vi "uc480_SimpleLive_MultiCamera.vi"() -> ()   [LabVIEW 2015]
uses:
  C:/Program Files/Thorlabs/Scientific Imaging/DCx Camera Support/Develop/DotNet/uc480DotNet.dll
panel:
  out "Image Out":T1(plugin-control)
  in  "Init Camera 2":bool
  in  "Exit Camera 2":bool
  out "Error Out 2":errorcluster caption="error"
  out "Bits/Pixel 2":i32=8
  out "Width":i32=8
  out "Height Height 2":i32=8
  out "Serial Number 2":string
  in  "Camera ID 2":i32
  out "Image second camera":picture
  out "Image first camera":picture
  in  "Camera ID 1":i32
  out "Serial Number 1":string
  out "Height Height":i32=8
  out "Width":i32=8
  out "Bits/Pixel":i32=8
  out "Error Out 1":errorcluster caption="error"
  in  "Exit Camera":bool
  in  "Init Camera":bool
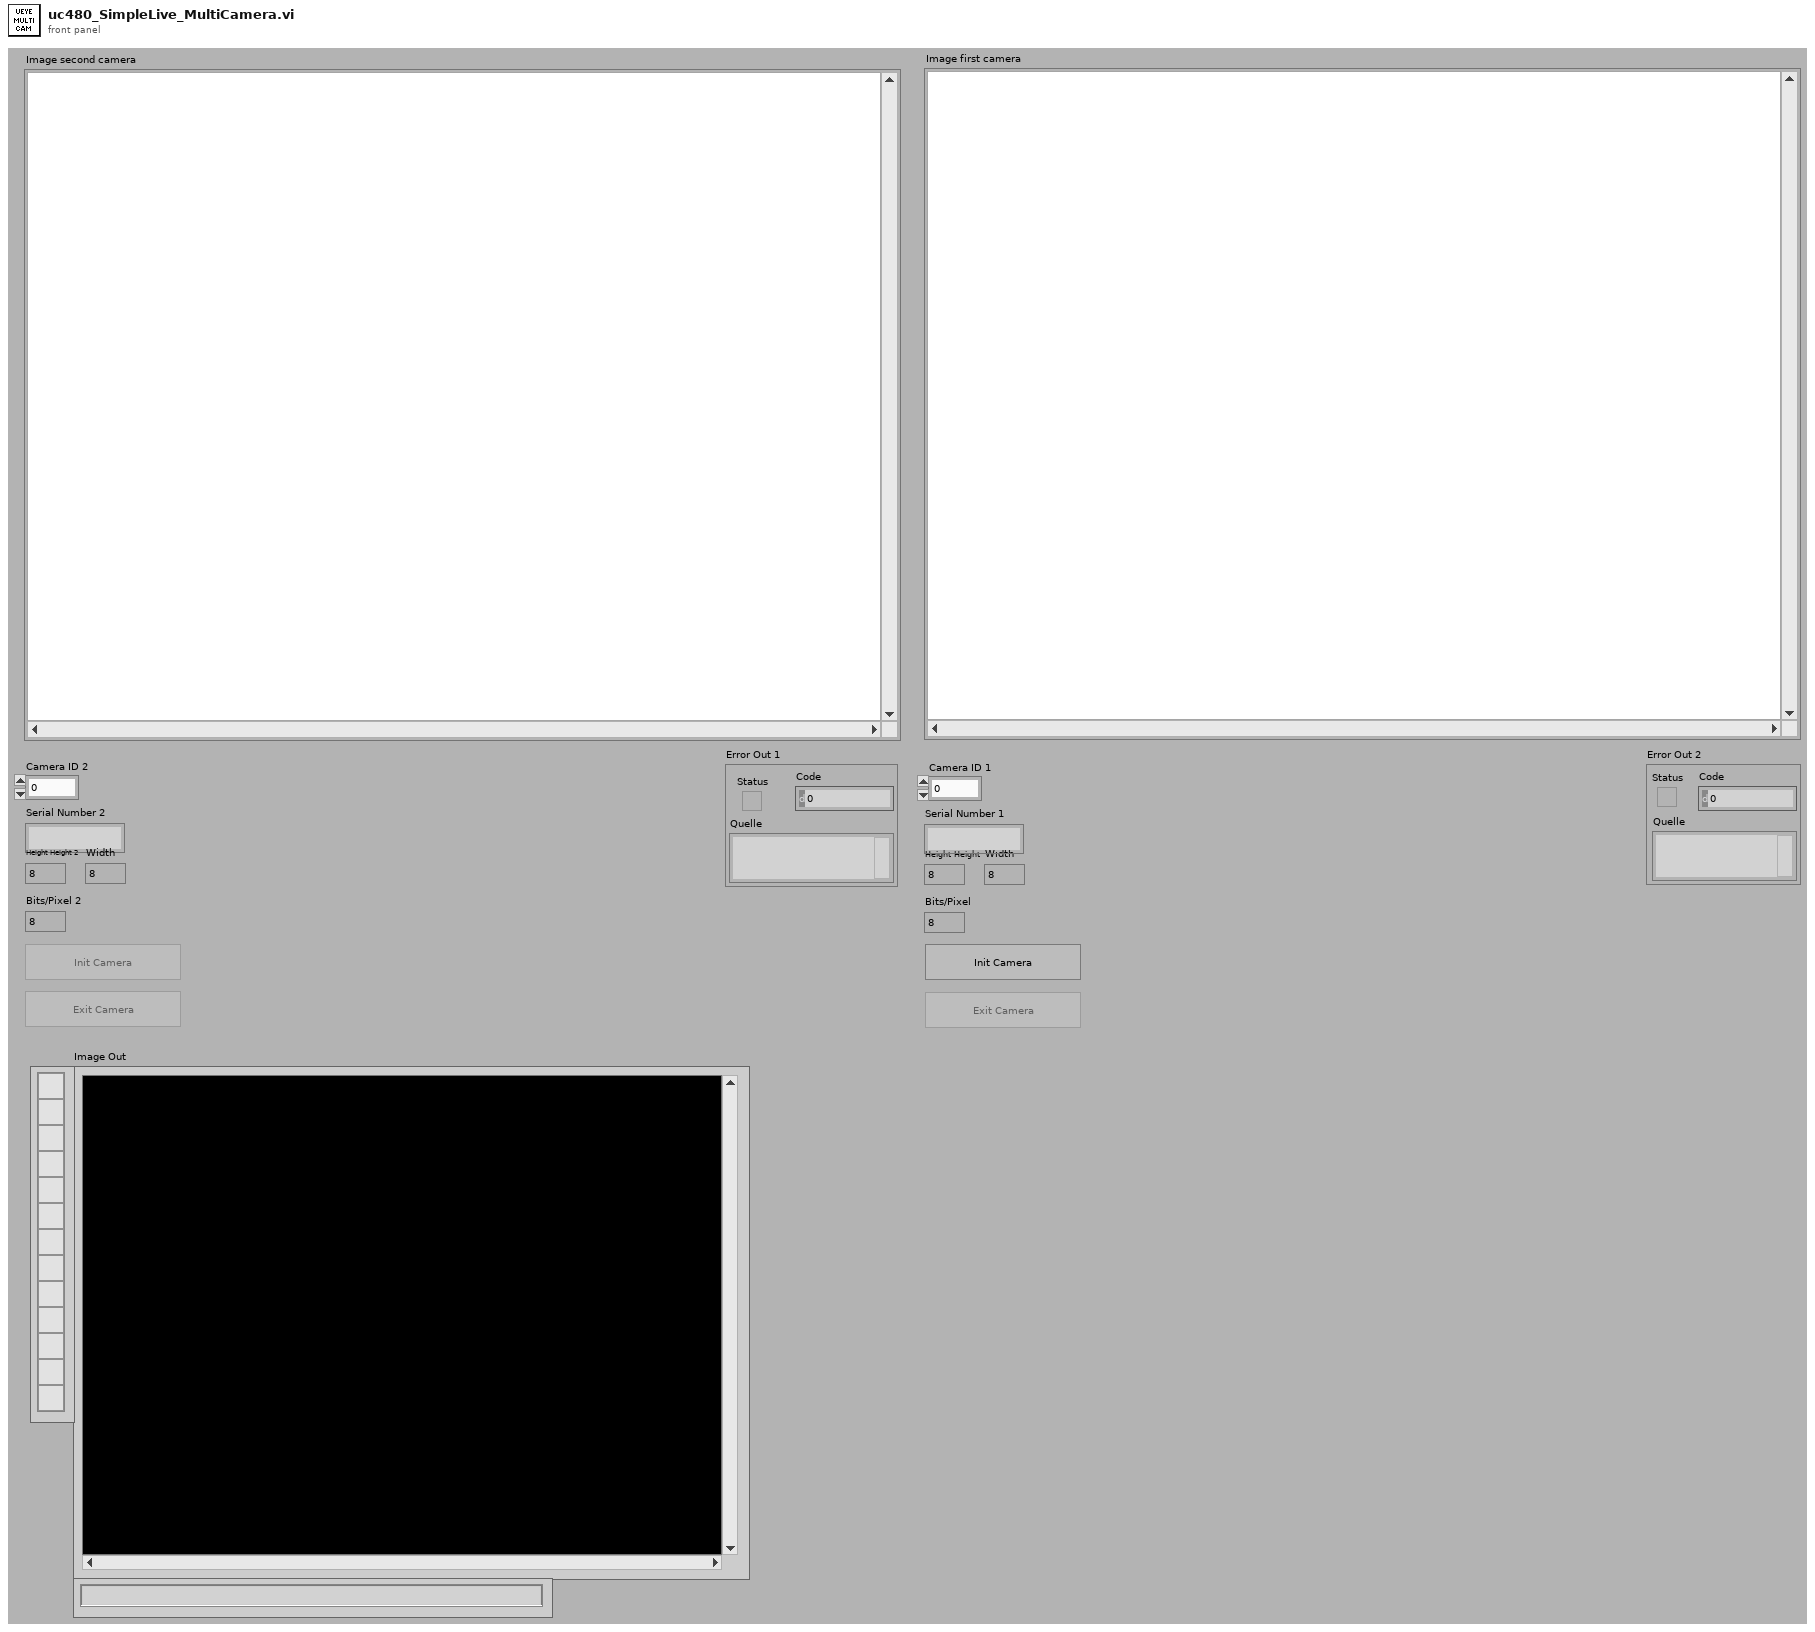
[diagram p1: front panel]
types:
  T1 = typedef "IMAQ Image.ctl" = refnum<image>
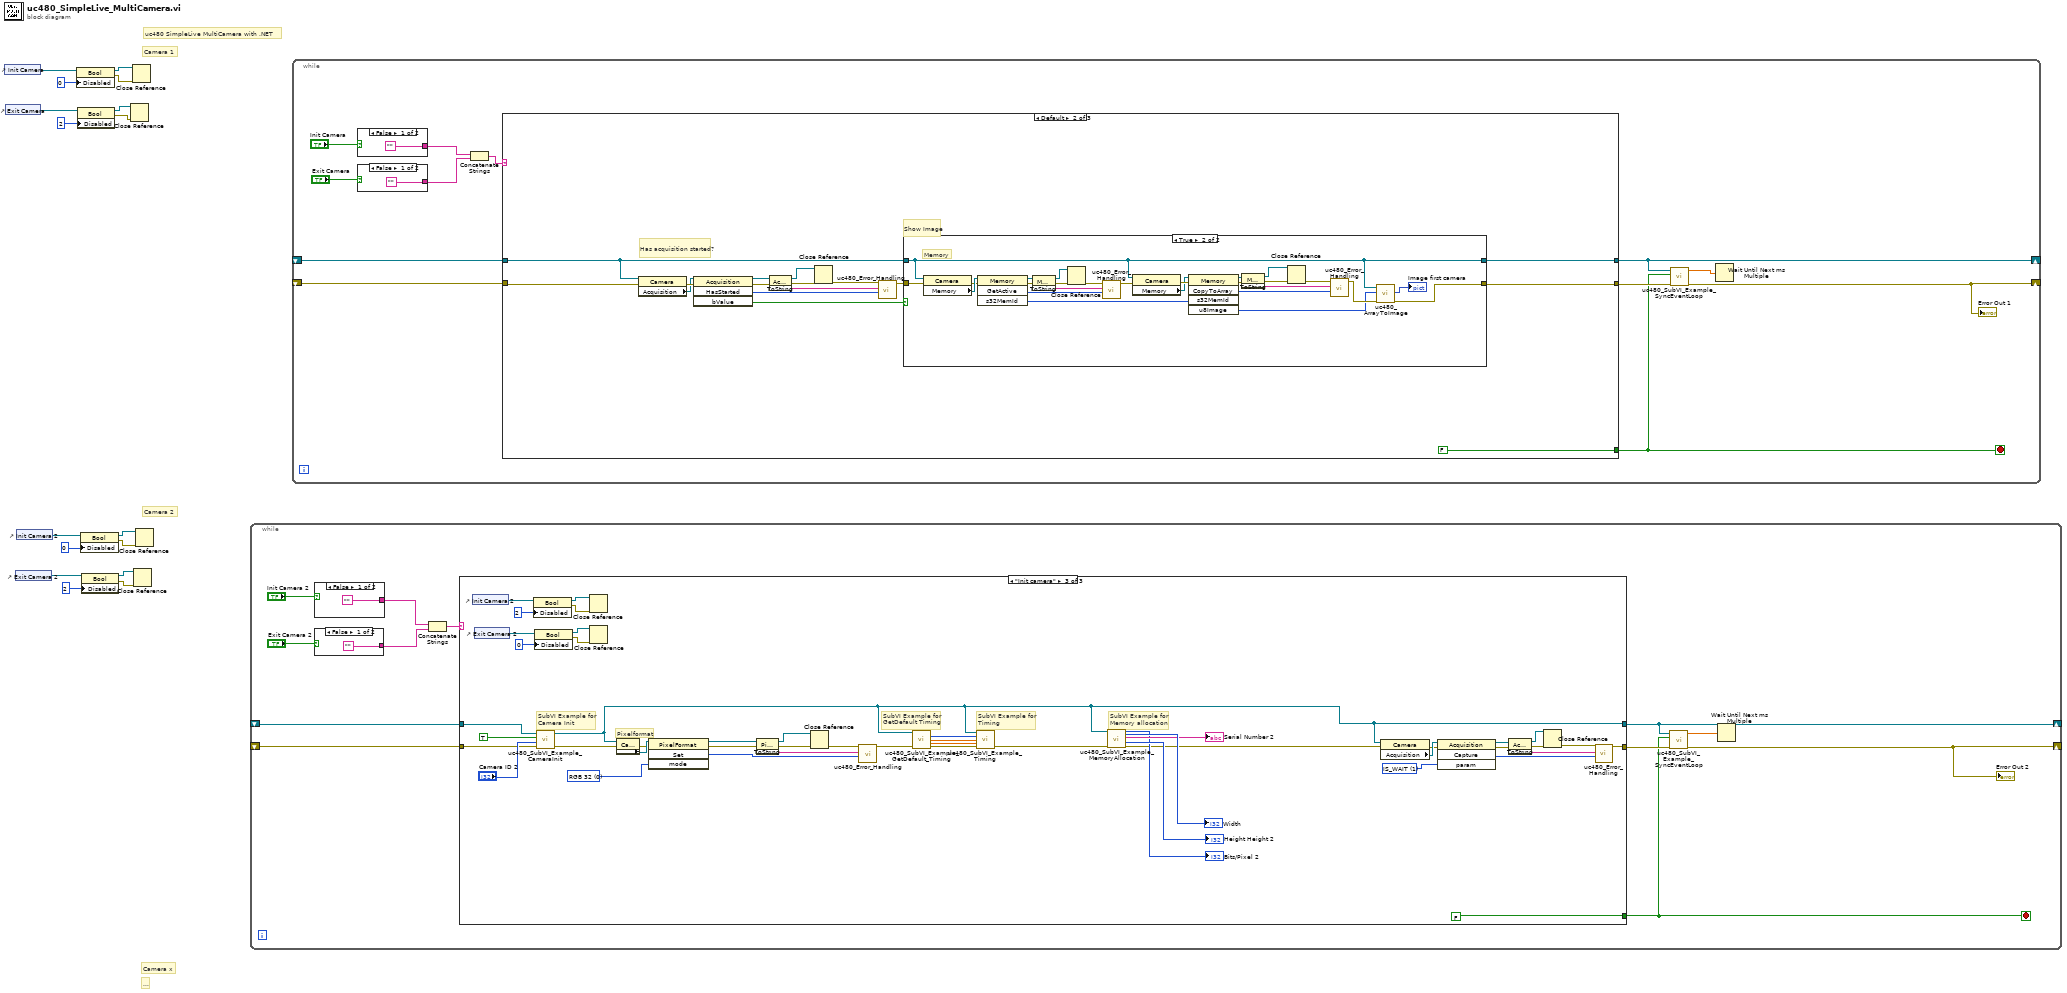
[diagram p0: block diagram]
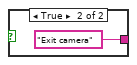
[diagram p2: hidden frame]
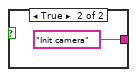
[diagram p3: hidden frame]
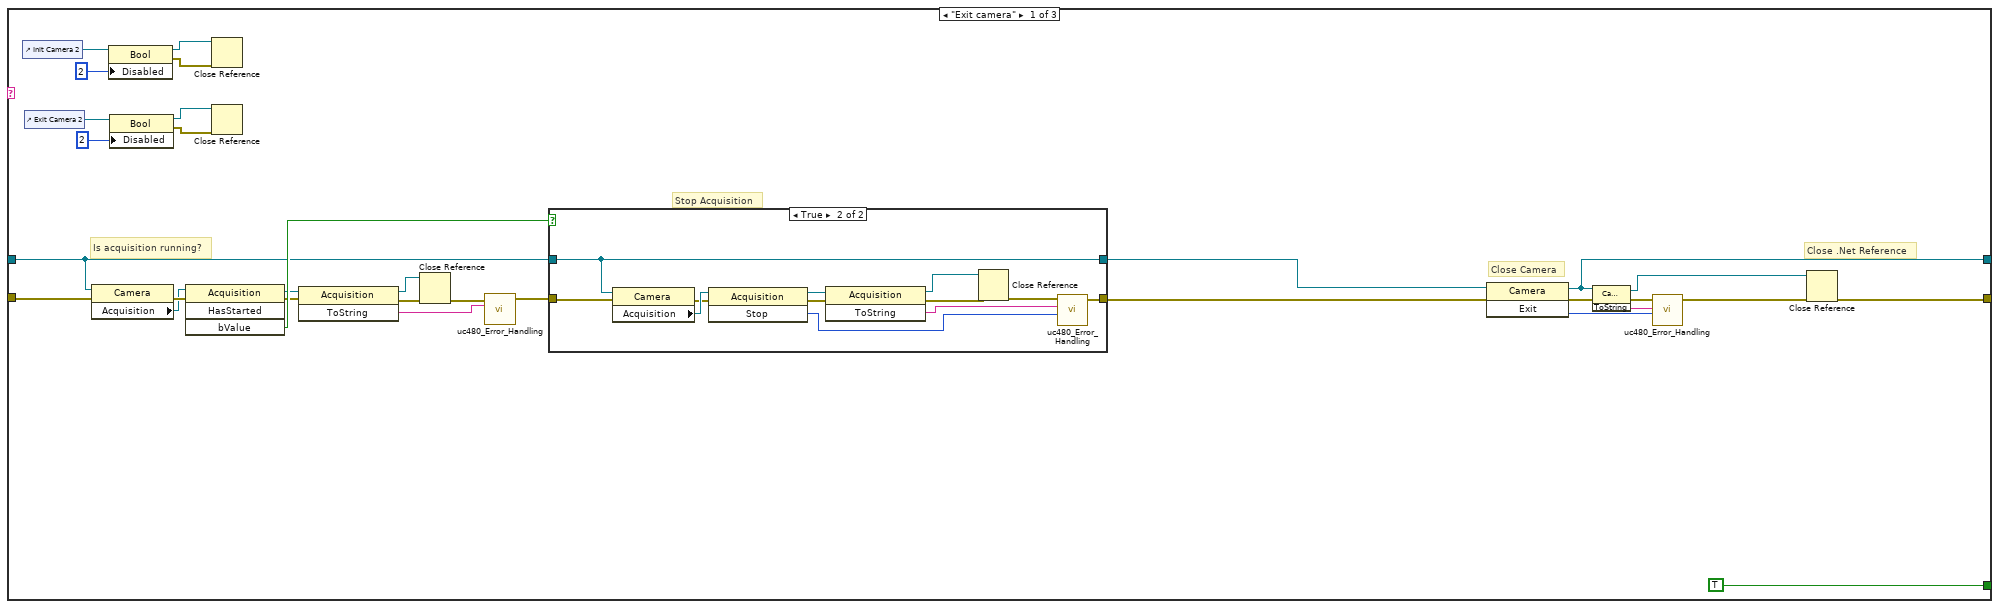
[diagram p4: hidden frame]
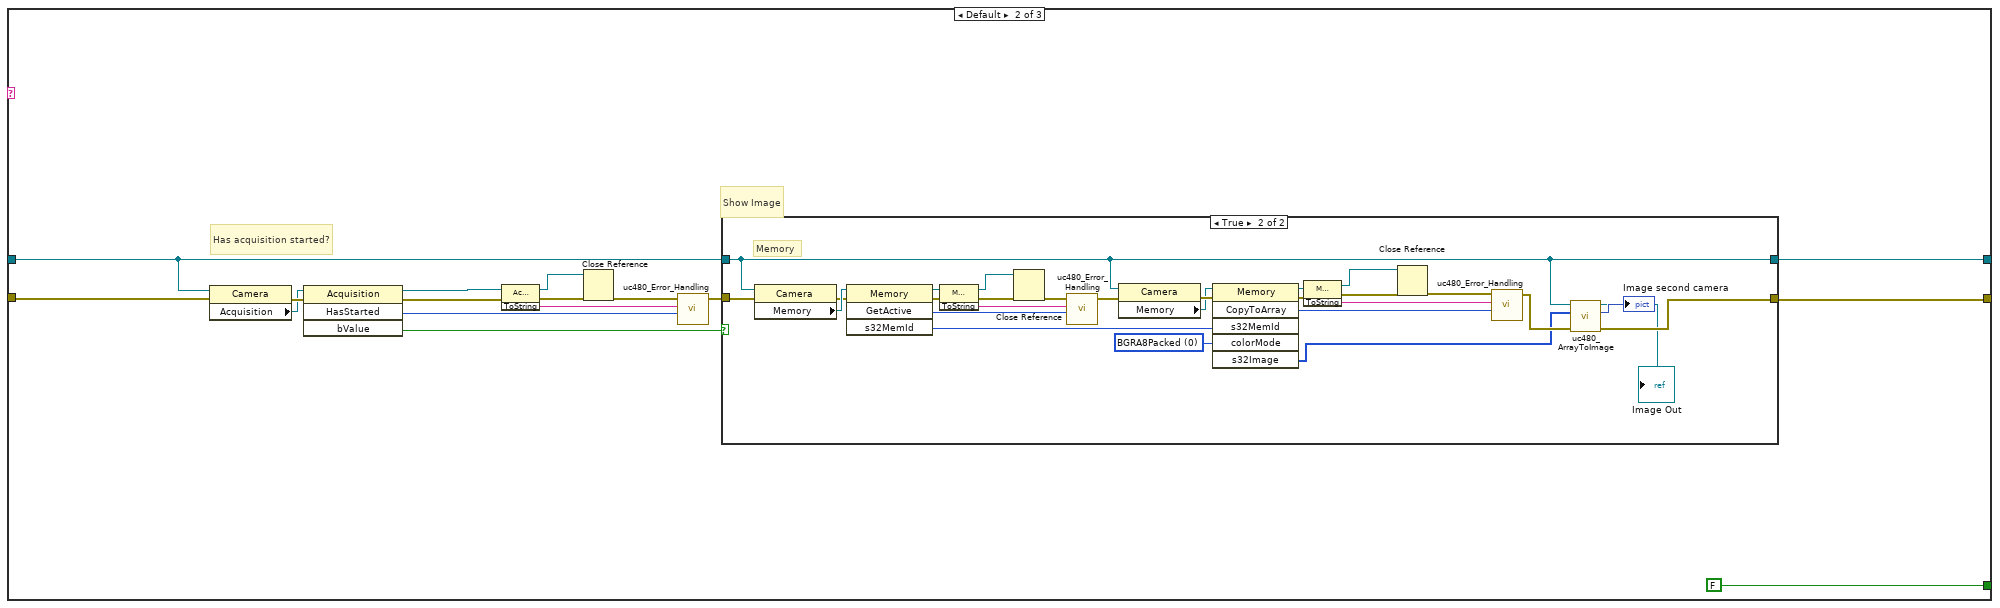
[diagram p6: hidden frame]
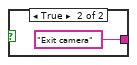
[diagram p8: hidden frame]
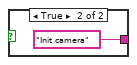
[diagram p9: hidden frame]
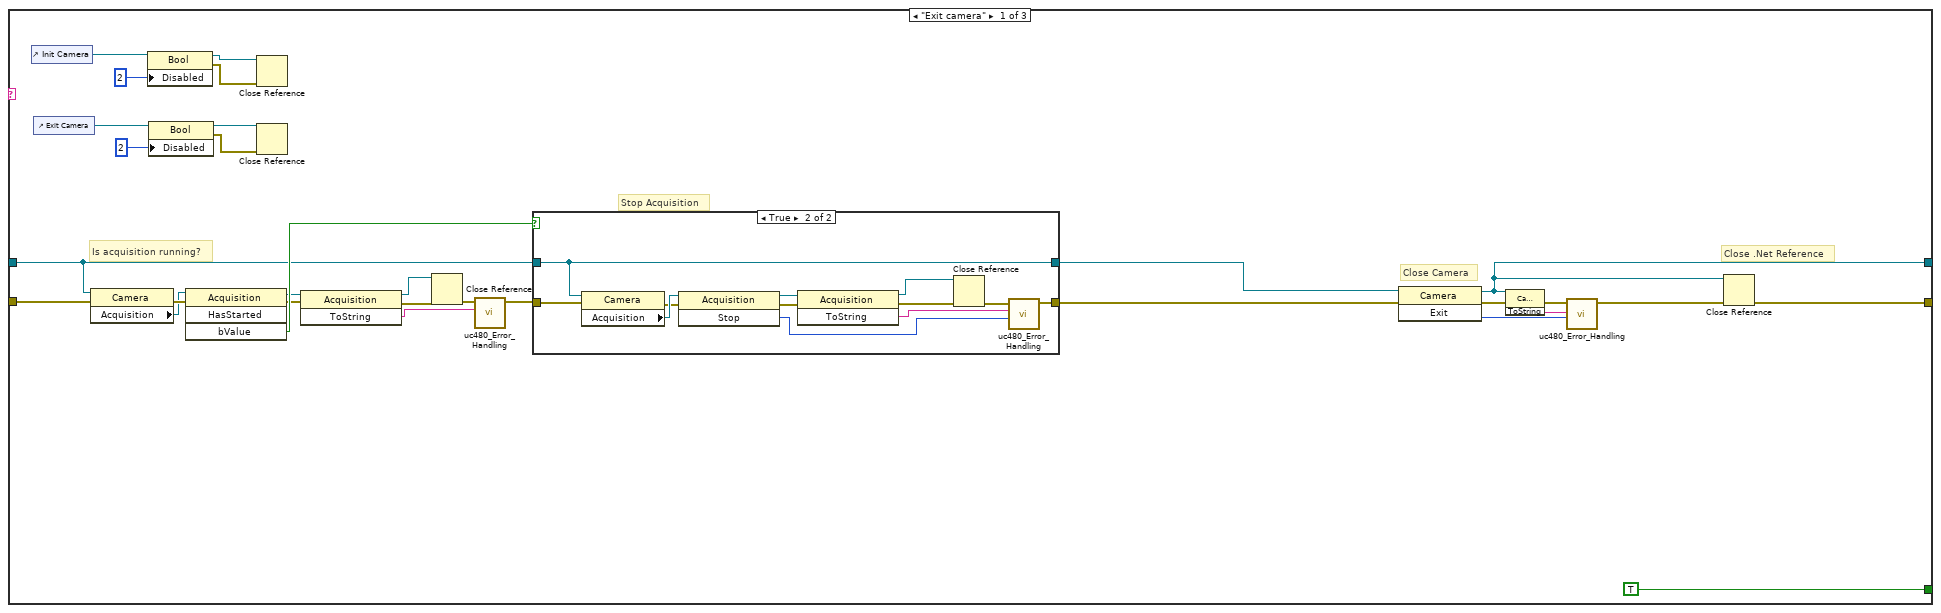
[diagram p10: hidden frame]
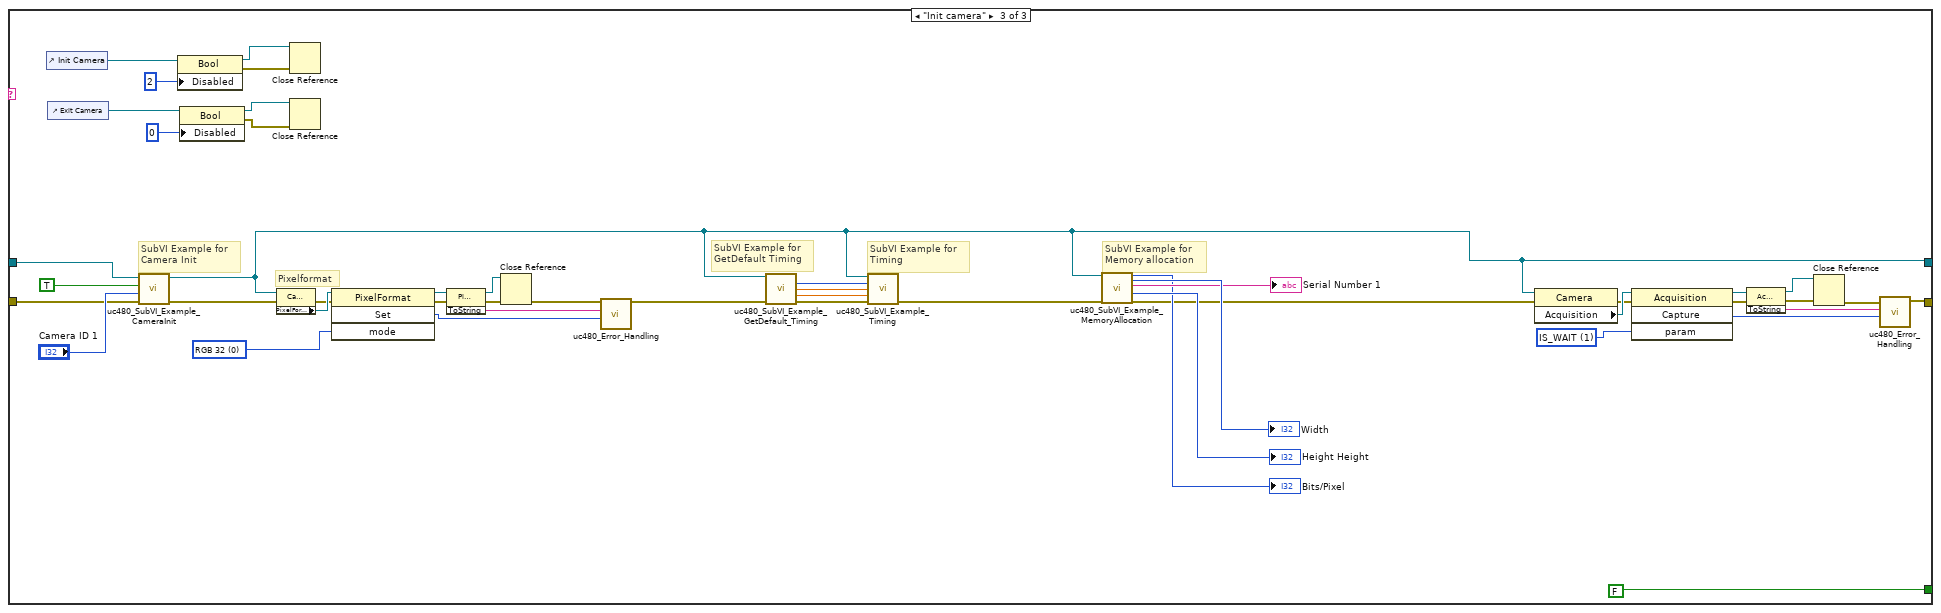
[diagram p13: hidden frame]
diagram:
  # "..."
  # "Camera x"
  # "Camera 2"
  # "Camera 1"
  # "uc480 SimpleLive MultiCamera with .NET"
  n1 = control-ref of="Init Camera"() -> (w14:refnum<vi>)
  n2 = control-ref of="Exit Camera"() -> (w13:refnum<vi>)
  n3 = control-ref of="Exit Camera 2"() -> (w9:refnum<vi>)
  n4 = control-ref of="Init Camera 2"() -> (w10:refnum<vi>)
  n5 = property class="Bool"(reference=w14, "Disabled"=u8 0 ("Deaktiviert")) -> (reference out=w8:refnum<vi>, error out=w7:errorcluster)  [unwired: 1 in]
  n6 = property class="Bool"(reference=w13, "Disabled"=u8 2 ("Deaktiviert")) -> (reference out=w6:refnum<vi>, error out=w5:errorcluster)  [unwired: 1 in]
  n7 = property class="Bool"(reference=w10, "Disabled"=u8 0 ("Deaktiviert")) -> (reference out=w4:refnum<vi>, error out=w3:errorcluster)  [unwired: 1 in]
  n8 = property class="Bool"(reference=w9, "Disabled"=u8 2 ("Deaktiviert")) -> (reference out=w2:refnum<vi>, error out=w1:errorcluster)  [unwired: 1 in]
  n9 = Close Reference ("Close Referenz")(reference=w6, error in (no error)=w5) -> ()  [unwired: 1 out]
  n10 = Close Reference ("Close Referenz")(reference=w8, error in (no error)=w7) -> ()  [unwired: 1 out]
  n11 = Close Reference ("Close Referenz")(reference=w2, error in (no error)=w1) -> ()  [unwired: 1 out]
  n12 = Close Reference ("Close Referenz")(reference=w4, error in (no error)=w3) -> ()  [unwired: 1 out]
  n13 = while {
    shift-right: [w19] -> _
    shift-left: _ -> [w23]
    shift-right: [w20] -> _
    shift-left: _ -> [w17]
    stop <- w18 stop-if-true
    n14 = case shown="False" "Exit Camera 2" {
      tunnel: ["" "Exit camera"] -> w24
      frame False {
      }
      frame True {
      }
    }
    n15 = case shown="False" "Init Camera 2" {
      tunnel: ["" "Init camera"] -> w27
      frame False {
      }
      frame True {
      }
    }
    n16 = Concatenate Strings(w27, w24) -> (w26:string)
    n17 = case shown="\"Init camera\"" w26 {
      tunnel: w17 -> [w47 w82 w162]
      tunnel: w23 -> [w48 w81 w161]
      tunnel: [w56 w84 w139] -> w20
      tunnel: [w57 w83 w140] -> w22
      tunnel: [TRUE FALSE FALSE] -> w18
      frame "Exit camera" {
        # "Close .Net Reference"
        # "Is acquisition running?"
        # "Stop Acquisition"
        # "Close Camera"
        n18 = control-ref of="Init Camera 2"() -> (w42:refnum<vi>)
        n19 = control-ref of="Exit Camera 2"() -> (w41:refnum<vi>)
        n20 = property class="Camera"(reference=w47, error in=w48) -> (error out=w55:errorcluster, "Acquisition"=w54:refnum<k24>)  [unwired: 1 out]
        n21 = property class="Bool"(reference=w42, "Disabled"=u8 2 ("Deaktiviert")) -> (reference out=w36:refnum<vi>, error out=w35:errorcluster)  [unwired: 1 in]
        n22 = property class="Bool"(reference=w41, "Disabled"=u8 2 ("Deaktiviert")) -> (reference out=w34:refnum<vi>, error out=w33:errorcluster)  [unwired: 1 in]
        n23 = invoke class="Acquisition" method="HasStarted"(reference=w54, error in=w55) -> (reference out=w49:refnum<k24>, error out=w51:errorcluster, "bValue"=w53:bool)  [unwired: 2 in, 1 out]
        n24 = Close Reference ("Close Referenz")(reference=w36, error in (no error)=w35) -> ()  [unwired: 1 out]
        n25 = Close Reference ("Close Referenz")(reference=w34, error in (no error)=w33) -> ()  [unwired: 1 out]
        n26 = invoke class="Acquisition" method="ToString"(reference=w49, error in=w51) -> (reference out=w37:refnum<k24>, error out=w39:errorcluster, "ToString"=w50:string)  [unwired: 1 in]
        n27 = Close Reference(reference=w37, error in (no error)=w39) -> (error out=w38:errorcluster)
        n28 = call "uc480_Error_Handling.vi"("Error String"=w50, "Error In"=w38) -> ("Error Out"=w52:errorcluster)  [unwired: 9 in]
        n29 = case shown="True" w53 {
          tunnel: [w65 w76] -> w45
          tunnel: w52 -> [w65 w77]
          tunnel: w47 -> [w64 w69]
          tunnel: [w64 w69] -> w46
          frame False {
          }
          frame True {
            n30 = property class="Camera"(reference=w69, error in=w77) -> (error out=w73:errorcluster, "Acquisition"=w74:refnum<k24>)  [unwired: 1 out]
            n31 = invoke class="Acquisition" method="Stop"(reference=w74, error in=w73) -> (reference out=w71:refnum<k24>, error out=w72:errorcluster, "Stop"=w70:i32)  [unwired: 1 in]
            n32 = invoke class="Acquisition" method="ToString"(reference=w71, error in=w72) -> (reference out=w66:refnum<k24>, error out=w68:errorcluster, "ToString"=w75:string)  [unwired: 1 in]
            n33 = Close Reference(reference=w66, error in (no error)=w68) -> (error out=w67:errorcluster)
            n34 = call "uc480_Error_Handling.vi"("Error Code"=w70, "Error String"=w75, "Error In"=w67) -> ("Error Out"=w76:errorcluster)  [unwired: 8 in]
          }
        }
        n35 = invoke class="Camera" method="Exit"(reference=w46, error in=w45) -> (reference out=w56:refnum<k24>, error out=w60:errorcluster, "Exit"=w59:i32)  [unwired: 1 in]
        n36 = invoke class="Camera" method="ToString"(reference=w56, error in=w60) -> (reference out=w40:refnum<k24>, error out=w61:errorcluster, "ToString"=w62:string)  [unwired: 1 in]
        n37 = call "uc480_Error_Handling.vi"("Error Code"=w59, "Error String"=w62, "Error In"=w61) -> ("Error Out"=w58:errorcluster)  [unwired: 8 in]
        n38 = Close Reference ("Close Referenz")(reference=w40, error in (no error)=w58) -> (error out=w57:errorcluster)
      }
      frame Default {
        # "Has acquisition started?"
        # "Show Image"
        n39 = property class="Camera"(reference=w82, error in=w81) -> (error out=w92:errorcluster, "Acquisition"=w91:refnum<k24>)  [unwired: 1 out]
        n40 = invoke class="Acquisition" method="HasStarted"(reference=w91, error in=w92) -> (reference out=w88:refnum<k24>, error out=w87:errorcluster, "HasStarted"=w86:i32, "bValue"=w90:bool)  [unwired: 2 in]
        n41 = invoke class="Acquisition" method="ToString"(reference=w88, error in=w87) -> (reference out=w78:refnum<k24>, error out=w80:errorcluster, "ToString"=w89:string)  [unwired: 1 in]
        n42 = Close Reference(reference=w78, error in (no error)=w80) -> (error out=w79:errorcluster)
        n43 = call "uc480_Error_Handling.vi"("Error Code"=w86, "Error String"=w89, "Error In"=w79) -> ("Error Out"=w85:errorcluster)  [unwired: 8 in]
        n44 = case shown="True" w90 {
          tunnel: [w95 w109] -> w83
          tunnel: w85 -> [w95 w108]
          tunnel: w82 -> [w94 w105]
          tunnel: [w94 w105] -> w84
          frame False {
          }
          frame True {
            w98 = 0 items=["BGRA8Packed"=0, "BGR8Packed"=1, "BGR565Packed"=2, "BGR5Packed"=3, "Mono8"=6, "SensorRaw8"=11, "UYVYPacked"=12, "UYVYMonoPacked"=13, "UYVYBayerPacked"=14, "CBYCRYPacked"=23, "BGRY8Packed"=24, "BGR10Packed"=25, "Mono12"=26, "SensorRaw12"=27, "Mono16"=28, "SensorRaw16"=29, "BGR12Unpacked"=30, "BGRA12Unpacked"=31, "Jpeg"=32, "SensorRaw10"=33, "Mono10"=34, "BGR10Unpacked"=35, "RGBA8Packed"=128, "RGB8Packed"=129, "RGBY8Packed"=152, "RGB10Packed"=153, "RGB12Unpacked"=158, "RGBA12Unpacked"=159, "RGB10Unpacked"=163, "RGB8Planar"=8321, "PreferPackedSourceFormat"=16384] ("colorMode")
            # "Memory"
            n45 = property class="Camera"(reference=w105, error in=w108) -> (error out=w111:errorcluster, "Memory"=w112:refnum<k24>)  [unwired: 1 out]
            n46 = invoke class="Memory" method="GetActive"(reference=w112, error in=w111) -> (reference out=w117:refnum<k24>, error out=w116:errorcluster, "GetActive"=w118:i32, "s32MemId"=w110:i32)  [unwired: 2 in]
            n47 = invoke class="Memory" method="ToString"(reference=w117, error in=w116) -> (reference out=w102:refnum<k24>, error out=w104:errorcluster, "ToString"=w115:string)  [unwired: 1 in]
            n48 = Close Reference(reference=w102, error in (no error)=w104) -> (error out=w103:errorcluster)
            n49 = call "uc480_Error_Handling.vi"("Error Code"=w118, "Error String"=w115, "Error In"=w103) -> ("Error Out"=w119:errorcluster)  [unwired: 8 in]
            n50 = property class="Camera"(reference=w105, error in=w119) -> (error out=w114:errorcluster, "Memory"=w113:refnum<k24>)  [unwired: 1 out]
            n51 = invoke class="Memory" method="CopyToArray"(reference=w113, error in=w114, "s32MemId"=w110, "colorMode"=w98) -> (reference out=w121:refnum<k24>, error out=w122:errorcluster, "CopyToArray"=w123:i32, "s32Image"=w97:i32[])  [unwired: 2 in, 2 out]
            n52 = invoke class="Memory" method="ToString"(reference=w121, error in=w122) -> (reference out=w99:refnum<k24>, error out=w101:errorcluster, "ToString"=w120:string)  [unwired: 1 in]
            n53 = Close Reference(reference=w99, error in (no error)=w101) -> (error out=w100:errorcluster)
            n54 = call "uc480_Error_Handling.vi"("Error Code"=w123, "Error String"=w120, "Error In"=w100) -> ("Error Out"=w106:errorcluster)  [unwired: 8 in]
            n55 = call "uc480_ArrayToImage.vi"("Error In"=w106, "InArray"=w97, ".NET (Reference)"=w105) -> ("Error Out"=w109:errorcluster, "Image"=→"Image second camera":picture, "Image Out"=→"Image Out":T1)  [unwired: 6 in]
          }
        }
      }
      frame "Init camera" {
        w141 = 1 items=["IS_DONT_WAIT", "IS_WAIT"] ("Wait")
        w170 = 0 items=["RGB 32"=0, "RGB 24"=1, "Y8 Monochrom"=6] ("Mode")
        # "SubVI Example for \nGetDefault Timing"
        # "SubVI Example for \nMemory allocation"
        # "SubVI Example for \nTiming"
        # "SubVI Example for \nCamera Init"
        # "Pixelformat"
        n56 = control-ref of="Init Camera 2"() -> (w136:refnum<vi>)
        n57 = control-ref of="Exit Camera 2"() -> (w134:refnum<vi>)
        n58 = property class="Bool"(reference=w136, "Disabled"=u8 2 ("Deaktiviert")) -> (reference out=w127:refnum<vi>, error out=w126:errorcluster)  [unwired: 1 in]
        n59 = property class="Bool"(reference=w134, "Disabled"=u8 0 ("Deaktiviert")) -> (reference out=w125:refnum<vi>, error out=w124:errorcluster)  [unwired: 1 in]
        n60 = call "uc480_SubVI_Example_CameraInit.vi"("Error In"=w161, "Camera ID"="Camera ID 2", "Init Camera Flag"=TRUE, ".NET (Reference)"=w162) -> ("Error Out"=w167:errorcluster, ".NET (Reference)"=w139:refnum<k24>)  [unwired: 6 in]
        n61 = Close Reference ("Close Referenz")(reference=w127, error in (no error)=w126) -> ()  [unwired: 1 out]
        n62 = Close Reference ("Close Referenz")(reference=w125, error in (no error)=w124) -> ()  [unwired: 1 out]
        n63 = property class="Camera"(reference=w139, error in=w167) -> (error out=w168:errorcluster, "PixelFormat"=w169:refnum<k24>)  [unwired: 1 out]
        n64 = invoke class="PixelFormat" method="Set"(reference=w169, error in=w168, "mode"=w170) -> (reference out=w165:refnum<k24>, error out=w158:errorcluster, "Set"=w164:i32)  [unwired: 1 in, 1 out]
        n65 = invoke class="PixelFormat" method="ToString"(reference=w165, error in=w158) -> (reference out=w131:refnum<k24>, error out=w133:errorcluster, "ToString"=w166:string)  [unwired: 1 in]
        n66 = Close Reference(reference=w131, error in (no error)=w133) -> (error out=w132:errorcluster)
        n67 = call "uc480_Error_Handling.vi"("Error Code"=w164, "Error String"=w166, "Error In"=w132) -> ("Error Out"=w152:errorcluster)  [unwired: 8 in]
        n68 = call "uc480_SubVI_Example_GetDefault_Timing.vi"(".NET (Reference)"=w139, "Error In"=w152) -> ("Pixelclock"=w149:i32, "Exposure time"=w150:dbl, "Framerate"=w151:dbl, "Error Out"=w148:errorcluster)  [unwired: 10 in]
        n69 = call "uc480_SubVI_Example_Timing.vi"(".NET (Reference)"=w139, "Pixelclock"=w149, "Exposure time"=w150, "Framerate"=w151, "Error In"=w148) -> ("Error Out"=w157:errorcluster)  [unwired: 7 in, 3 out]
        n70 = call "uc480_SubVI_Example_MemoryAllocation.vi"(".NET (Reference)"=w139, "Error In"=w157) -> ("Bits/Pixel 2"=→"Bits/Pixel 2":i32, "Width"=→"Width":i32, "Serial Number"=→"Serial Number 2":string, "Height"=→"Height Height 2":i32, "Error Out"=w138:errorcluster)  [unwired: 13 in]
        n71 = property class="Camera"(reference=w139, error in=w138) -> (error out=w146:errorcluster, "Acquisition"=w147:refnum<k24>)  [unwired: 1 out]
        n72 = invoke class="Acquisition" method="Capture"(reference=w147, error in=w146, "param"=w141) -> (reference out=w143:refnum<k24>, error out=w144:errorcluster, "Capture"=w142:i32)  [unwired: 1 in, 1 out]
        n73 = invoke class="Acquisition" method="ToString"(reference=w143, error in=w144) -> (reference out=w128:refnum<k24>, error out=w130:errorcluster, "ToString"=w145:string)  [unwired: 1 in]
        n74 = Close Reference(reference=w128, error in (no error)=w130) -> (error out=w129:errorcluster)
        n75 = call "uc480_Error_Handling.vi"("Error Code"=w142, "Error String"=w145, "Error In"=w129) -> ("Error Out"=w140:errorcluster)  [unwired: 8 in]
      }
    }
    n76 = call "uc480_SubVI_Example_SyncEventLoop.vi"("Error In"=w22, "use sync"=w18, ".NET (Reference)"=w20) -> ("Error Out"=w19:errorcluster, "Synchronize (ms)"=w21:dbl)  [unwired: 7 in]
    "Error Out 2" <- w19
    n77 = Wait Until Next ms Multiple(millisecond multiple=w21) -> ()  [unwired: 1 out]
  }
  n78 = while {
    shift-right: [w174] -> _
    shift-left: _ -> [w177]
    shift-right: [w175] -> _
    shift-left: _ -> [w171]
    stop <- w172 stop-if-true
    n79 = case shown="False" "Init Camera" {
      tunnel: ["" "Init camera"] -> w181
      frame False {
      }
      frame True {
      }
    }
    n80 = case shown="False" "Exit Camera" {
      tunnel: ["" "Exit camera"] -> w178
      frame False {
      }
      frame True {
      }
    }
    n81 = Concatenate Strings(w181, w178) -> (w180:string)
    n82 = case shown="Default" w180 {
      tunnel: w171 -> [w200 w235 w313]
      tunnel: w177 -> [w201 w234 w312]
      tunnel: [w209 w237 w291] -> w175
      tunnel: [w210 w236 w292] -> w176
      tunnel: [TRUE FALSE FALSE] -> w172
      frame "Exit camera" {
        # "Close .Net Reference"
        # "Is acquisition running?"
        # "Stop Acquisition"
        # "Close Camera"
        n83 = control-ref of="Init Camera"() -> (w195:refnum<vi>)
        n84 = control-ref of="Exit Camera"() -> (w194:refnum<vi>)
        n85 = property class="Camera"(reference=w200, error in=w201) -> (error out=w208:errorcluster, "Acquisition"=w207:refnum<k24>)  [unwired: 1 out]
        n86 = property class="Bool"(reference=w195, "Disabled"=u8 2 ("Deaktiviert")) -> (reference out=w190:refnum<vi>, error out=w189:errorcluster)  [unwired: 1 in]
        n87 = property class="Bool"(reference=w194, "Disabled"=u8 2 ("Deaktiviert")) -> (reference out=w188:refnum<vi>, error out=w187:errorcluster)  [unwired: 1 in]
        n88 = invoke class="Acquisition" method="HasStarted"(reference=w207, error in=w208) -> (reference out=w202:refnum<k24>, error out=w204:errorcluster, "bValue"=w206:bool)  [unwired: 2 in, 1 out]
        n89 = Close Reference ("Close Referenz")(reference=w190, error in (no error)=w189) -> ()  [unwired: 1 out]
        n90 = Close Reference ("Close Referenz")(reference=w188, error in (no error)=w187) -> ()  [unwired: 1 out]
        n91 = invoke class="Acquisition" method="ToString"(reference=w202, error in=w204) -> (reference out=w191:refnum<k24>, error out=w193:errorcluster, "ToString"=w203:string)  [unwired: 1 in]
        n92 = Close Reference(reference=w191, error in (no error)=w193) -> (error out=w192:errorcluster)
        n93 = call "uc480_Error_Handling.vi"("Error String"=w203, "Error In"=w192) -> ("Error Out"=w205:errorcluster)  [unwired: 9 in]
        n94 = case shown="True" w206 {
          tunnel: [w218 w229] -> w198
          tunnel: w205 -> [w218 w230]
          tunnel: w200 -> [w217 w222]
          tunnel: [w217 w222] -> w199
          frame False {
          }
          frame True {
            n95 = property class="Camera"(reference=w222, error in=w230) -> (error out=w226:errorcluster, "Acquisition"=w227:refnum<k24>)  [unwired: 1 out]
            n96 = invoke class="Acquisition" method="Stop"(reference=w227, error in=w226) -> (reference out=w224:refnum<k24>, error out=w225:errorcluster, "Stop"=w223:i32)  [unwired: 1 in]
            n97 = invoke class="Acquisition" method="ToString"(reference=w224, error in=w225) -> (reference out=w219:refnum<k24>, error out=w221:errorcluster, "ToString"=w228:string)  [unwired: 1 in]
            n98 = Close Reference(reference=w219, error in (no error)=w221) -> (error out=w220:errorcluster)
            n99 = call "uc480_Error_Handling.vi"("Error Code"=w223, "Error String"=w228, "Error In"=w220) -> ("Error Out"=w229:errorcluster)  [unwired: 8 in]
          }
        }
        n100 = invoke class="Camera" method="Exit"(reference=w199, error in=w198) -> (reference out=w209:refnum<k24>, error out=w213:errorcluster, "Exit"=w212:i32)  [unwired: 1 in]
        n101 = invoke class="Camera" method="ToString"(reference=w209, error in=w213) -> (error out=w214:errorcluster, "ToString"=w215:string)  [unwired: 1 in, 1 out]
        n102 = call "uc480_Error_Handling.vi"("Error Code"=w212, "Error String"=w215, "Error In"=w214) -> ("Error Out"=w211:errorcluster)  [unwired: 8 in]
        n103 = Close Reference ("Close Referenz")(reference=w209, error in (no error)=w211) -> (error out=w210:errorcluster)
      }
      frame Default {
        # "Has acquisition started?"
        # "Show Image"
        n104 = property class="Camera"(reference=w235, error in=w234) -> (error out=w245:errorcluster, "Acquisition"=w244:refnum<k24>)  [unwired: 1 out]
        n105 = invoke class="Acquisition" method="HasStarted"(reference=w244, error in=w245) -> (reference out=w241:refnum<k24>, error out=w240:errorcluster, "HasStarted"=w239:i32, "bValue"=w243:bool)  [unwired: 2 in]
        n106 = invoke class="Acquisition" method="ToString"(reference=w241, error in=w240) -> (reference out=w231:refnum<k24>, error out=w233:errorcluster, "ToString"=w242:string)  [unwired: 1 in]
        n107 = Close Reference(reference=w231, error in (no error)=w233) -> (error out=w232:errorcluster)
        n108 = call "uc480_Error_Handling.vi"("Error Code"=w239, "Error String"=w242, "Error In"=w232) -> ("Error Out"=w238:errorcluster)  [unwired: 8 in]
        n109 = case shown="True" w243 {
          tunnel: [w248 w260] -> w236
          tunnel: w238 -> [w248 w259]
          tunnel: w235 -> [w247 w257]
          tunnel: [w247 w257] -> w237
          frame False {
          }
          frame True {
            # "Memory"
            n110 = property class="Camera"(reference=w257, error in=w259) -> (error out=w262:errorcluster, "Memory"=w263:refnum<k24>)  [unwired: 1 out]
            n111 = invoke class="Memory" method="GetActive"(reference=w263, error in=w262) -> (reference out=w268:refnum<k24>, error out=w267:errorcluster, "GetActive"=w269:i32, "s32MemId"=w261:i32)  [unwired: 2 in]
            n112 = invoke class="Memory" method="ToString"(reference=w268, error in=w267) -> (reference out=w252:refnum<k24>, error out=w254:errorcluster, "ToString"=w266:string)  [unwired: 1 in]
            n113 = Close Reference(reference=w252, error in (no error)=w254) -> (error out=w253:errorcluster)
            n114 = call "uc480_Error_Handling.vi"("Error Code"=w269, "Error String"=w266, "Error In"=w253) -> ("Error Out"=w270:errorcluster)  [unwired: 8 in]
            n115 = property class="Camera"(reference=w257, error in=w270) -> (error out=w265:errorcluster, "Memory"=w264:refnum<k24>)  [unwired: 1 out]
            n116 = invoke class="Memory" method="CopyToArray"(reference=w264, error in=w265, "s32MemId"=w261) -> (reference out=w272:refnum<k24>, error out=w273:errorcluster, "CopyToArray"=w274:i32, "u8Image"=w256:u8[])  [unwired: 2 in, 1 out]
            n117 = invoke class="Memory" method="ToString"(reference=w272, error in=w273) -> (reference out=w249:refnum<k24>, error out=w251:errorcluster, "ToString"=w271:string)  [unwired: 1 in]
            n118 = Close Reference(reference=w249, error in (no error)=w251) -> (error out=w250:errorcluster)
            n119 = call "uc480_Error_Handling.vi"("Error Code"=w274, "Error String"=w271, "Error In"=w250) -> ("Error Out"=w258:errorcluster)  [unwired: 8 in]
            n120 = call "uc480_ArrayToImage.vi"("Error In"=w258, "InArray"=w256, ".NET (Reference)"=w257) -> ("Error Out"=w260:errorcluster, "Image"=→"Image first camera":picture)  [unwired: 6 in, 1 out]
          }
        }
      }
      frame "Init camera" {
        w293 = 1 items=["IS_DONT_WAIT", "IS_WAIT"] ("Wait")
        w321 = 0 items=["RGB 32"=0, "RGB 24"=1, "Y8 Monochrom"=6] ("Mode")
        # "SubVI Example for \nGetDefault Timing"
        # "SubVI Example for \nMemory allocation"
        # "SubVI Example for \nTiming"
        # "SubVI Example for \nCamera Init"
        # "Pixelformat"
        n121 = control-ref of="Init Camera"() -> (w287:refnum<vi>)
        n122 = control-ref of="Exit Camera"() -> (w285:refnum<vi>)
        n123 = call "uc480_SubVI_Example_CameraInit.vi"("Error In"=w312, "Camera ID"="Camera ID 1", "Init Camera Flag"=TRUE, ".NET (Reference)"=w313) -> ("Error Out"=w318:errorcluster, ".NET (Reference)"=w291:refnum<k24>)  [unwired: 6 in]
        n124 = property class="Bool"(reference=w287, "Disabled"=u8 2 ("Deaktiviert")) -> (reference out=w278:refnum<vi>, error out=w277:errorcluster)  [unwired: 1 in]
        n125 = property class="Bool"(reference=w285, "Disabled"=u8 0 ("Deaktiviert")) -> (reference out=w276:refnum<vi>, error out=w275:errorcluster)  [unwired: 1 in]
        n126 = property class="Camera"(reference=w291, error in=w318) -> (error out=w319:errorcluster, "PixelFormat"=w320:refnum<k24>)  [unwired: 1 out]
        n127 = Close Reference ("Close Referenz")(reference=w278, error in (no error)=w277) -> ()  [unwired: 1 out]
        n128 = Close Reference ("Close Referenz")(reference=w276, error in (no error)=w275) -> ()  [unwired: 1 out]
        n129 = invoke class="PixelFormat" method="Set"(reference=w320, error in=w319, "mode"=w321) -> (reference out=w316:refnum<k24>, error out=w309:errorcluster, "Set"=w315:i32)  [unwired: 1 in, 1 out]
        n130 = invoke class="PixelFormat" method="ToString"(reference=w316, error in=w309) -> (reference out=w283:refnum<k24>, error out=w284:errorcluster, "ToString"=w317:string)  [unwired: 1 in]
        n131 = Close Reference(reference=w283, error in (no error)=w284) -> (error out=w282:errorcluster)
        n132 = call "uc480_Error_Handling.vi"("Error Code"=w315, "Error String"=w317, "Error In"=w282) -> ("Error Out"=w303:errorcluster)  [unwired: 8 in]
        n133 = call "uc480_SubVI_Example_GetDefault_Timing.vi"(".NET (Reference)"=w291, "Error In"=w303) -> ("Pixelclock"=w300:i32, "Exposure time"=w301:dbl, "Framerate"=w302:dbl, "Error Out"=w289:errorcluster)  [unwired: 10 in]
        n134 = call "uc480_SubVI_Example_Timing.vi"(".NET (Reference)"=w291, "Pixelclock"=w300, "Exposure time"=w301, "Framerate"=w302, "Error In"=w289) -> ("Error Out"=w308:errorcluster)  [unwired: 7 in, 3 out]
        n135 = call "uc480_SubVI_Example_MemoryAllocation.vi"(".NET (Reference)"=w291, "Error In"=w308) -> ("Bits/Pixel 2"=→"Bits/Pixel":i32, "Width"=→"Width":i32, "Serial Number"=→"Serial Number 1":string, "Height"=→"Height Height":i32, "Error Out"=w290:errorcluster)  [unwired: 13 in]
        n136 = property class="Camera"(reference=w291, error in=w290) -> (error out=w298:errorcluster, "Acquisition"=w299:refnum<k24>)  [unwired: 1 out]
        n137 = invoke class="Acquisition" method="Capture"(reference=w299, error in=w298, "param"=w293) -> (reference out=w295:refnum<k24>, error out=w296:errorcluster, "Capture"=w294:i32)  [unwired: 1 in, 1 out]
        n138 = invoke class="Acquisition" method="ToString"(reference=w295, error in=w296) -> (reference out=w279:refnum<k24>, error out=w281:errorcluster, "ToString"=w297:string)  [unwired: 1 in]
        n139 = Close Reference(reference=w279, error in (no error)=w281) -> (error out=w280:errorcluster)
        n140 = call "uc480_Error_Handling.vi"("Error Code"=w294, "Error String"=w297, "Error In"=w280) -> ("Error Out"=w292:errorcluster)  [unwired: 8 in]
      }
    }
    n141 = call "uc480_SubVI_Example_SyncEventLoop.vi"("Error In"=w176, "use sync"=w172, ".NET (Reference)"=w175) -> ("Error Out"=w174:errorcluster, "Synchronize (ms)"=w173:dbl)  [unwired: 7 in]
    "Error Out 1" <- w174
    n142 = Wait Until Next ms Multiple(millisecond multiple=w173) -> ()  [unwired: 1 out]
  }
